vi "THz_TimeDelay.vi"(8 "error in (no error)":errorcluster, 11 "Transport":refnum<class "Transport.lvclass">) -> (0 "error out":errorcluster, 3 "Transport out":refnum<class "Transport.lvclass">)   [LabVIEW 2019, in "Transport.lvclass"]
uses:
  Transport.lvclass
  Control Experiment/Control Experiment.lvclass
  <vilib>/measure/NI_MAPro.lvlib
  <vilib>/PRIrvin/XY Utilities/xy_utilities.lvlib
  <vilib>/PRIrvin/XY Utilities/subVIs/Waveform to XY (single).vi
  <vilib>/PRIrvin/XY Utilities/subVIs/Get X and Y (single).vi
  <vilib>/measure/maspectr.llb/FFT Power Spectrum and PSD for 1 Chan.vi
  <userlib>/_MGI/Timing/MGI Wait/MGI Wait (U32).vi
  <vilib>/Waveform/WDTOps.llb/WDT Append Waveforms DBL.vi
  <userlib>/LevyLab/Lockin-Multichannel/Instrument.Lockin/Instrument.Lockin.lvclass
  <userlib>/LevyLab/Instrument Framework/Instrument Types/Cryostat/Instrument.Cryostat.lvclass
  <userlib>/LevyLab/Instrument Framework/Instrument Types/Delay Line/Instrument.DelayLine.lvclass
  <userlib>/LevyLab/Instrument Framework/Instrument Types/Lockin/Instrument.LockinAPI.lvclass
  89c60be8-115d-42a4-a854-67badb4f6eec.vi
  C:/Program Files/National Instruments/LabVIEW 2019/user.lib/LevyLab/Instrument Framework/Instrument Types/Lockin/Instrument.LockinAPI.lvclass
  <vilib>/measure/maresamp.llb/Resample Pair of Arrays (single shot).vi
panel:
  out "Horizontal Progress Bar":dbl(slide)=0.5013000000000001 scale=-0.5..0.5
  out "Signal vs Time":T1(graph)
  out "Delay vs Time":cluster{"Time":dbl[], "Delay":dbl[]}(graph)
  out "Power Spectrum":cluster{"f0":dbl, "df":dbl, "magnitude":dbl[]}[](graph) caption="Power spectrum of time domain signal"
  in  "stop":bool
  out "Experiment Comments":string="describe only the experiment you're doing right now"
  out "Experiment Folder":string="05 - folder name"
  out "Delay (ps)":dbl
  out "Elapsed Time (s)":u32
  out "T (mK)":dbl
  out "Refresh Time (ms)":u32
  in  "Sweep Time (s)":dbl=10.0 format="%#_3p"
  in  "Initial Wait (s)":u32=1
  in  "Delay End (ps)":dbl=0.5
  in  "Delay Start (ps)":dbl=-0.5
  in  "Fs (S/s)":dbl=1000.0 min=1000.0 max=204800.0 format="%#_13g"
  in  "Lockin Refresh (s)":dbl=2.0
  in  "Timeout (ms)":i32=1000
  out "Current State":string="Exit"
  # "Start"
  # "End"
  # "*Change these values in Transport Server"
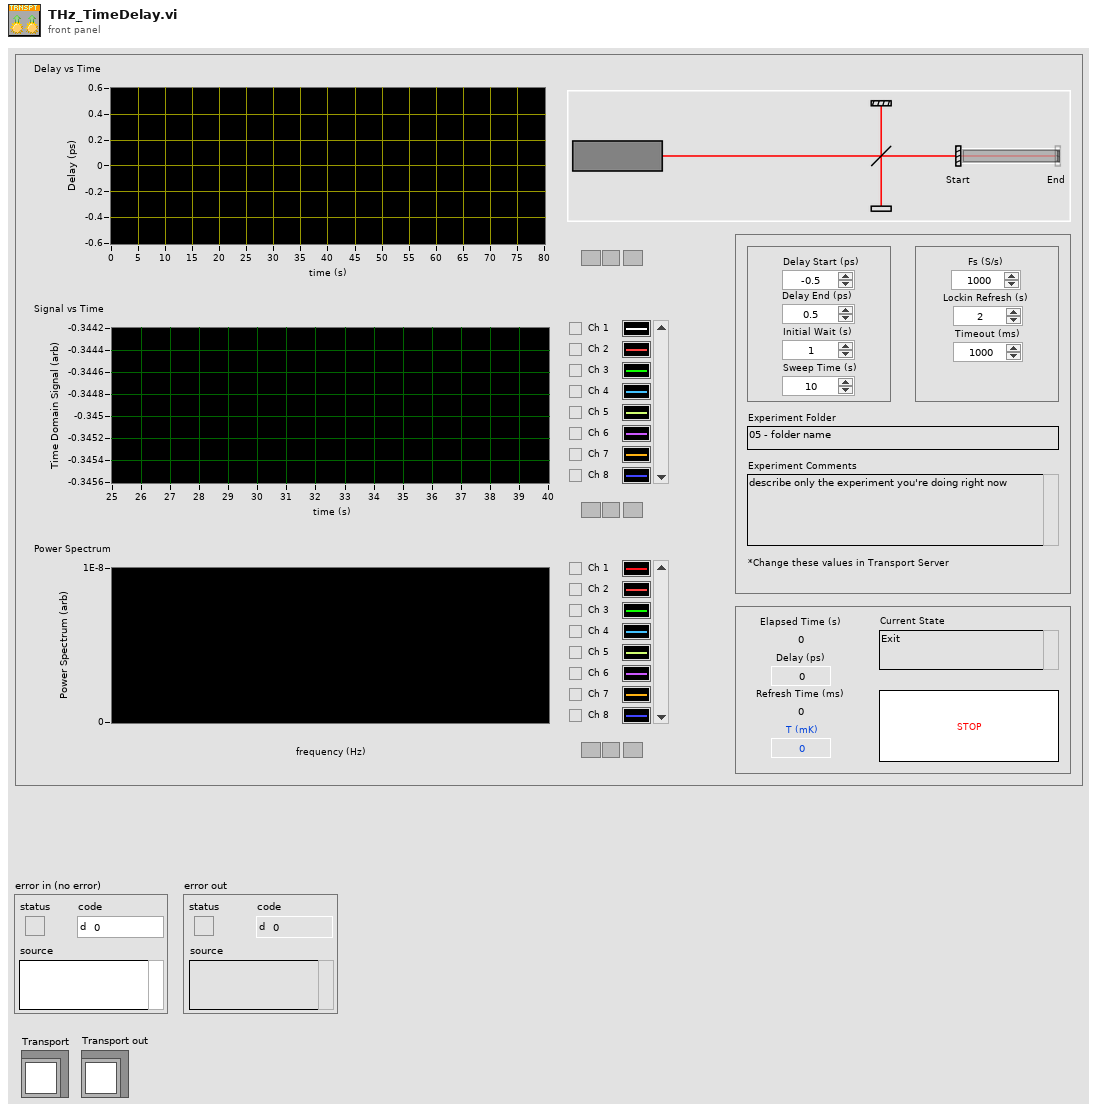
[diagram p1: front panel]
types:
  T1 = cluster{"Delay Start (ps)":dbl, dbl, "Y":dbl[]}[]
  T2 = enum32{"Invalid", "Standard", "Closed", "Hidden", "Minimized", "Maximized"}
  T3 = enum32{"invalid app kind", "Development System", "Run Time System", "Student Edition", "Embedded LabVIEW", "Evaluation", "Custom"}
  T4 = typedef "Control Experiment.lvclass/Instrument Classes--cluster.ctl" = cluster{"DAQ":refnum<class "Instrument.LockinAPI.lvclass">, "Amplifier":refnum<class "Instrument.Amplifier.lvclass">, "Temperature":refnum<class "Instrument.Cryostat.lvclass">, "Magnet":refnum<class "Instrument.Cryostat.lvclass">, "Rotator":refnum<class "Instrument.Cryostat.lvclass">, "Level":refnum<class "Instrument.Cryostat.lvclass">, "Capacitance":refnum<class "Instrument.CBridge.lvclass">, "Delay Line":refnum<class "Instrument.DelayLine.lvclass">, "Strain Cell":refnum<class "Instrument.Strain.lvclass">, "VNA":refnum<class "Instrument.VNA.lvclass">, "Source":refnum<class "Instrument.VSource.lvclass">}
  T5 = cluster{"Core":cluster{"Current VI Reference":refnum<vi>, "Close Panel on Exit?":bool}, "Transport":refnum<class "Transport.lvclass">, "C.E.":refnum<class "Control Experiment.lvclass">, "Instruments":T4, "Elapsed Time":dbl[], "Absolute Time":dbl[], "Temperature":dbl, "Magnet":dbl, "Delay":dbl[], "AI Waveform (s)":waveform(dbl)[], "AI Waveform (ps)":waveform(dbl)[], "t0":timestamp, "Sweep Value":dbl[], "ms [0]":u32, "ms [i]":u32, "Delay Range (ps)":dbl, "Delay Speed (ps/s)":dbl, "reset":bool, "delay line finish?":bool, "Execution:State":enum32{"Bad", "Idle", "Run top level", "Running"}}
  T6 = enum32{"Bad", "Idle", "Run top level", "Running"}
  T7 = cluster{"Current VI Reference":refnum<vi>, "Close Panel on Exit?":bool}
  T8 = typedef "Instrument.LockinAPI.lvclass/LockinAPI.Sampling.Sampling--Cluster.ctl" = cluster{"Fs":dbl, "#s":i32}
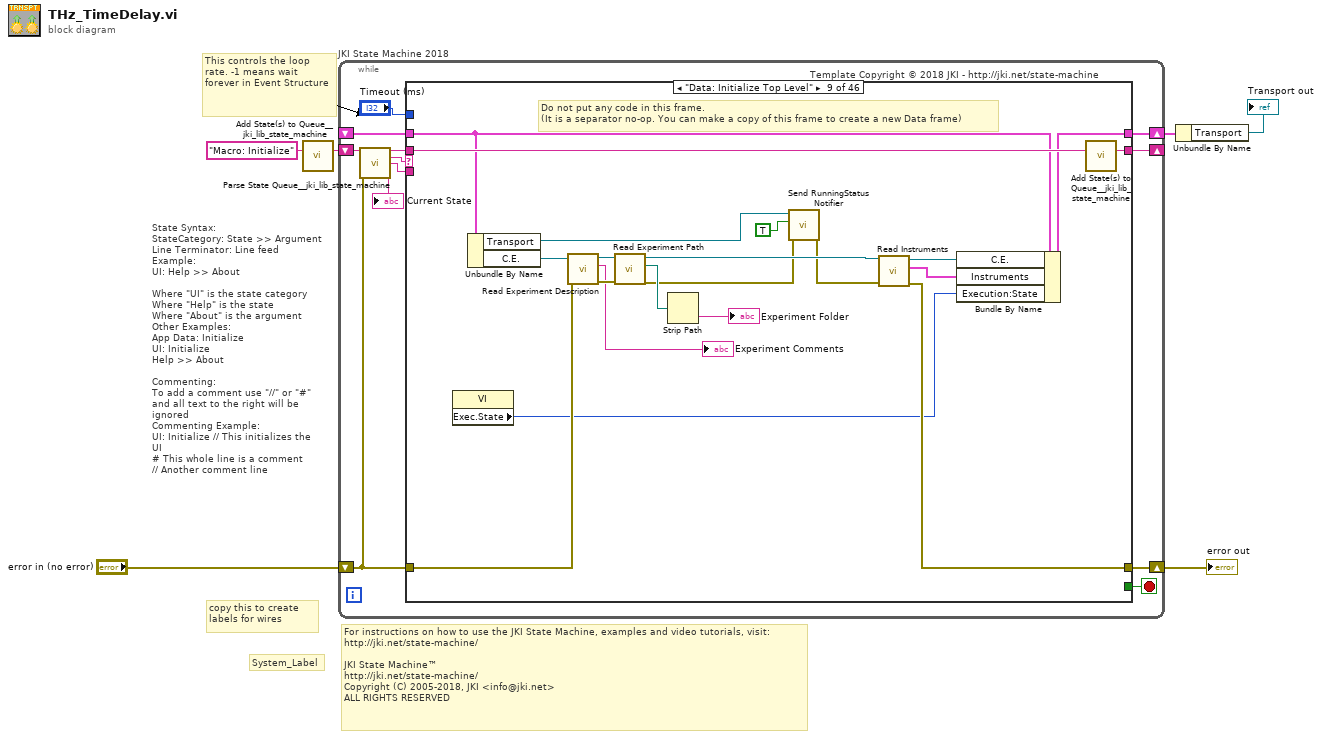
[diagram p0: block diagram]
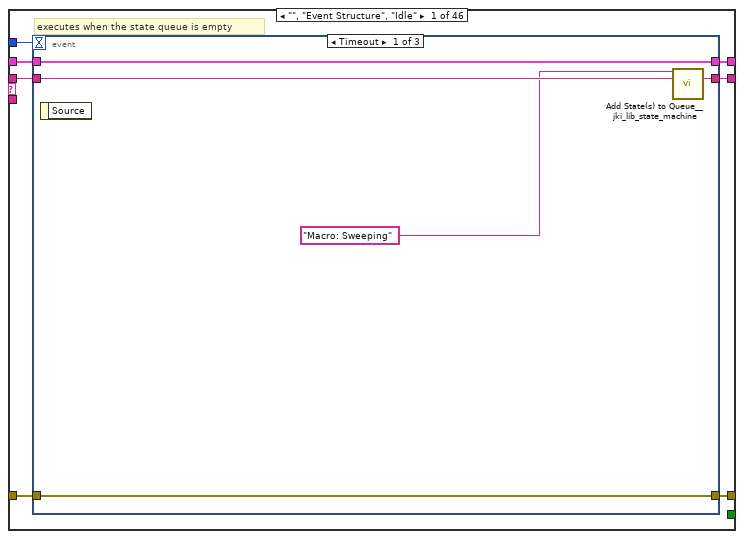
[diagram p2: hidden frame]
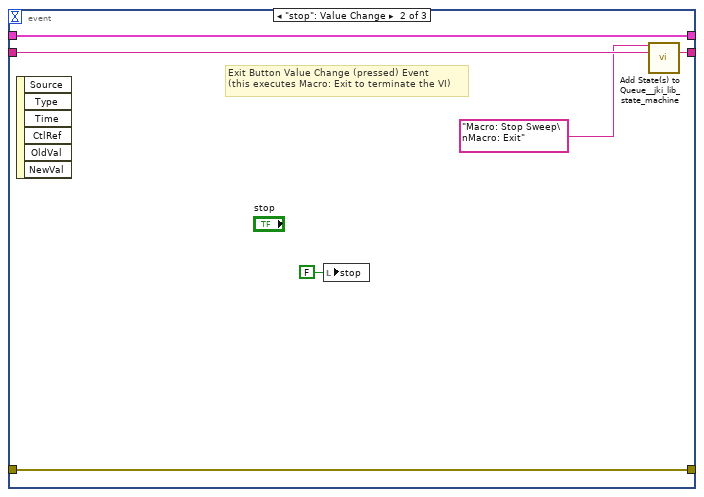
[diagram p3: hidden frame]
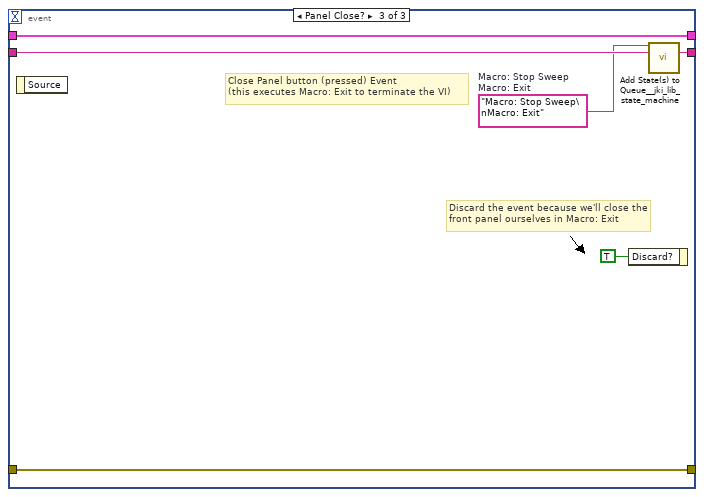
[diagram p4: hidden frame]
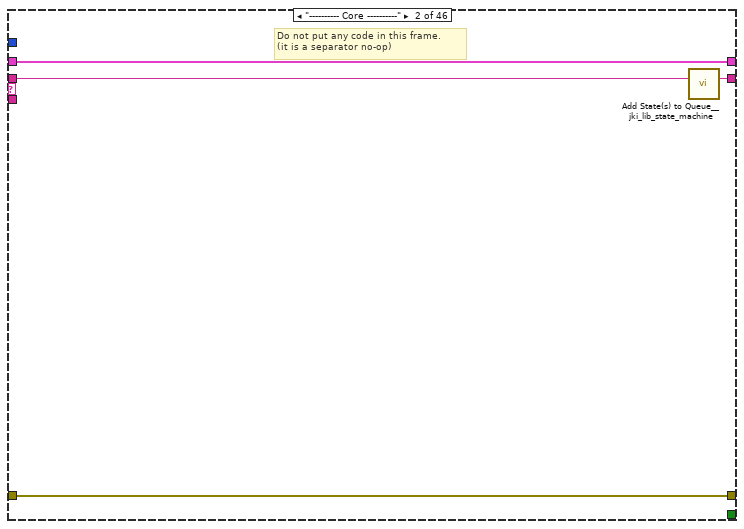
[diagram p5: hidden frame]
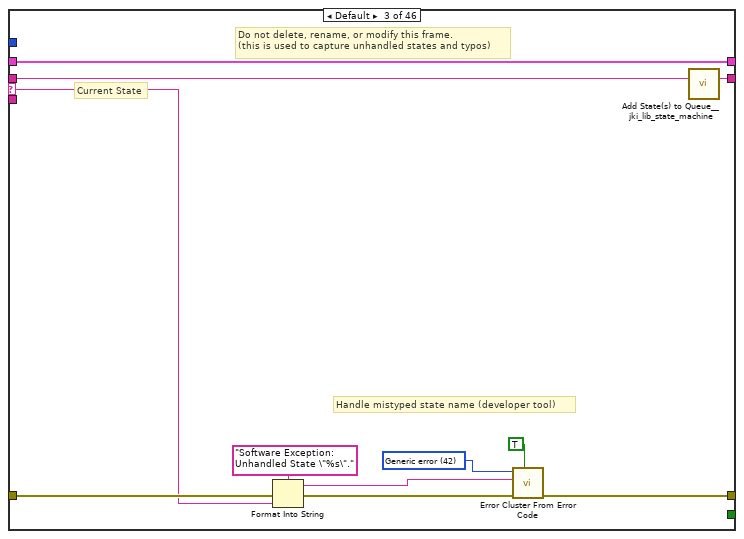
[diagram p6: hidden frame]
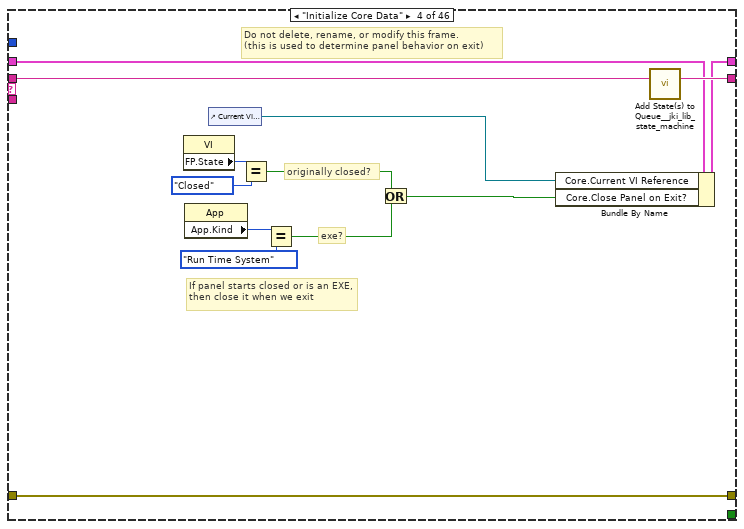
[diagram p7: hidden frame]
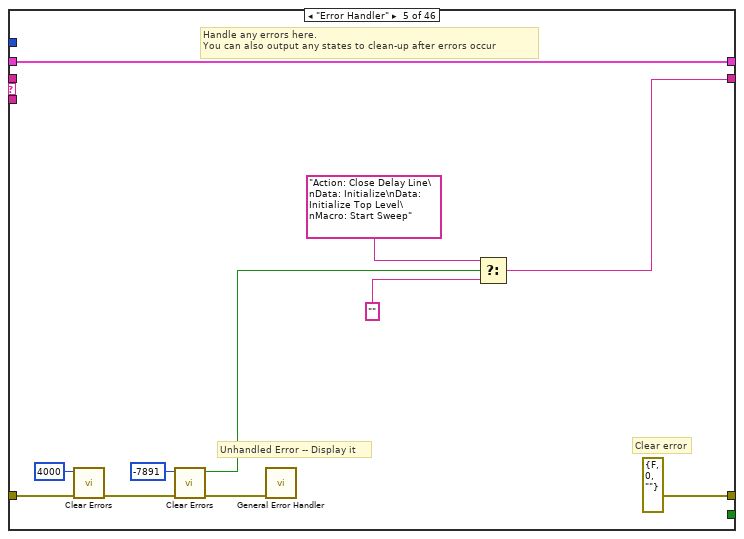
[diagram p8: hidden frame]
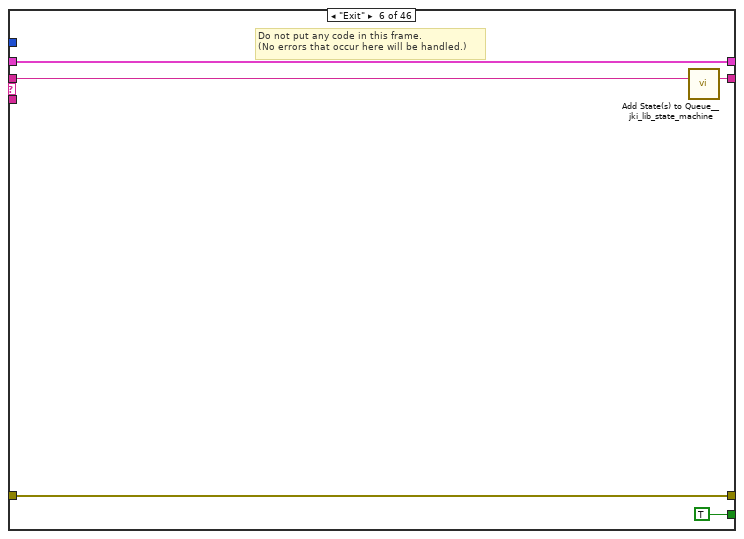
[diagram p9: hidden frame]
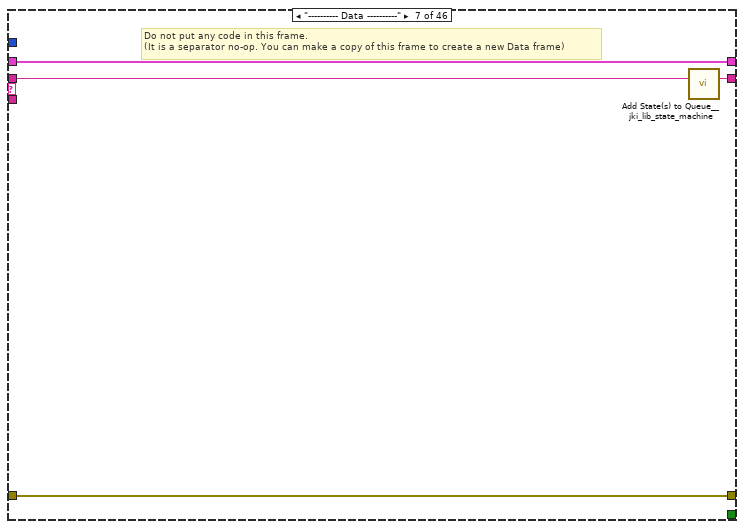
[diagram p10: hidden frame]
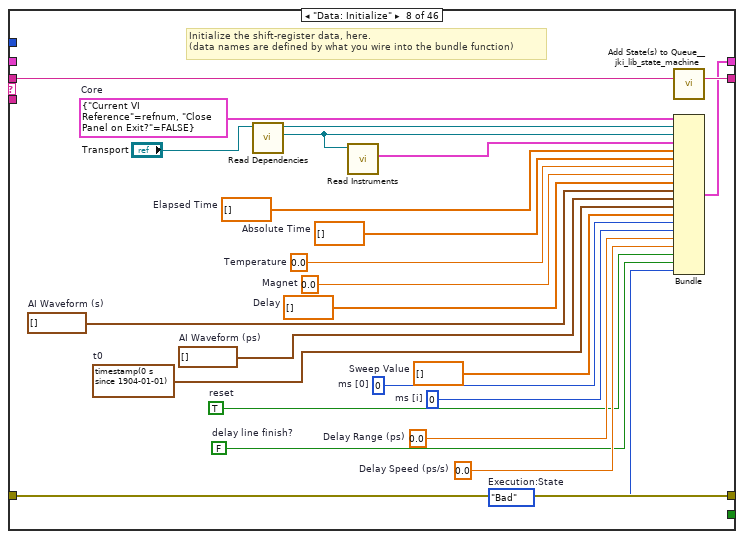
[diagram p11: hidden frame]
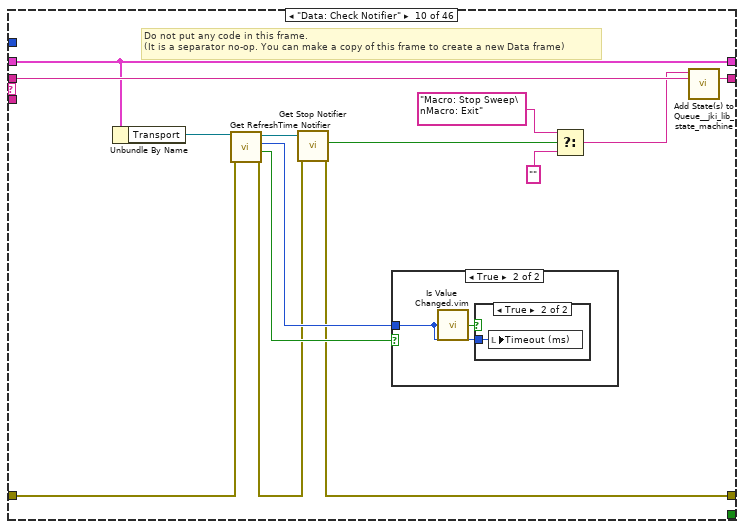
[diagram p12: hidden frame]
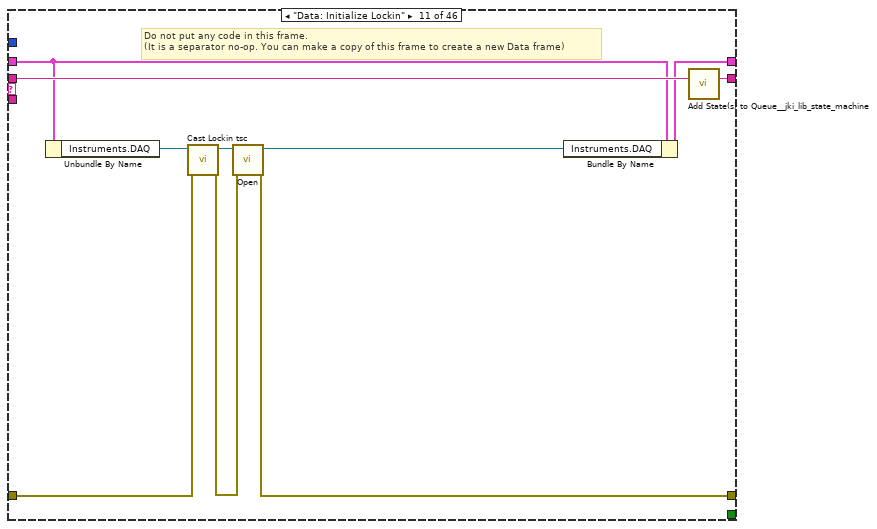
[diagram p15: hidden frame]
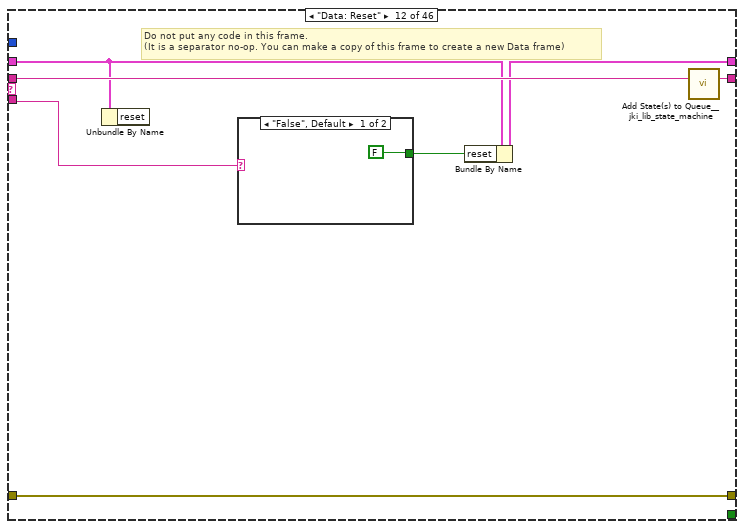
[diagram p16: hidden frame]
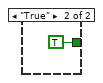
[diagram p17: hidden frame]
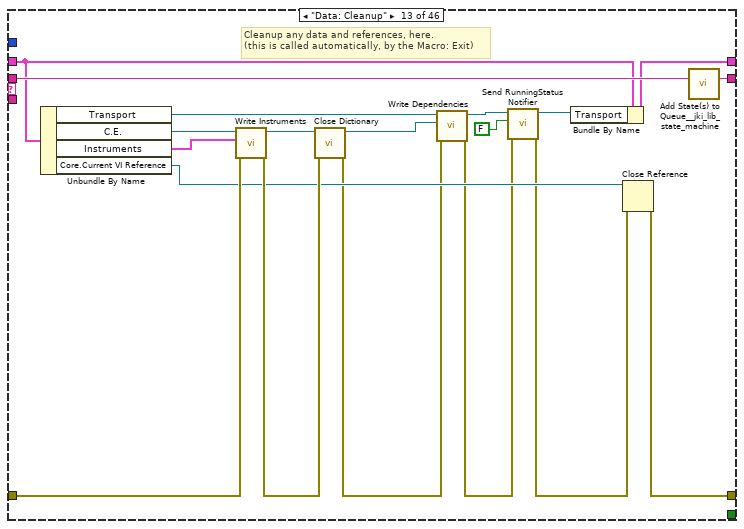
[diagram p18: hidden frame]
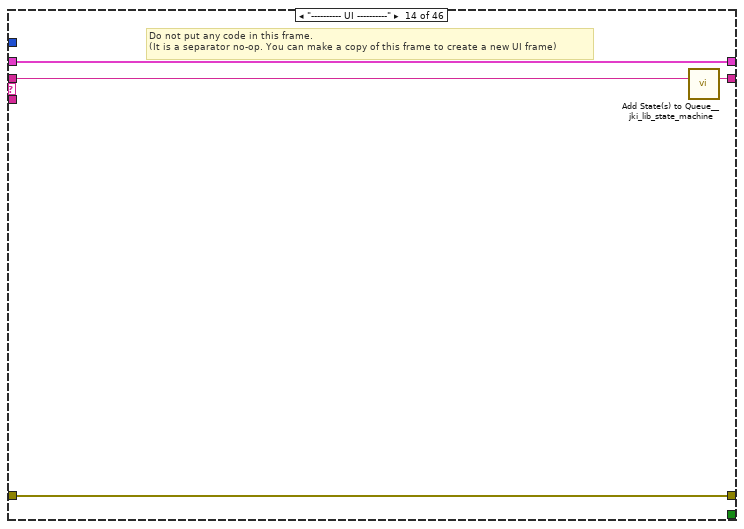
[diagram p19: hidden frame]
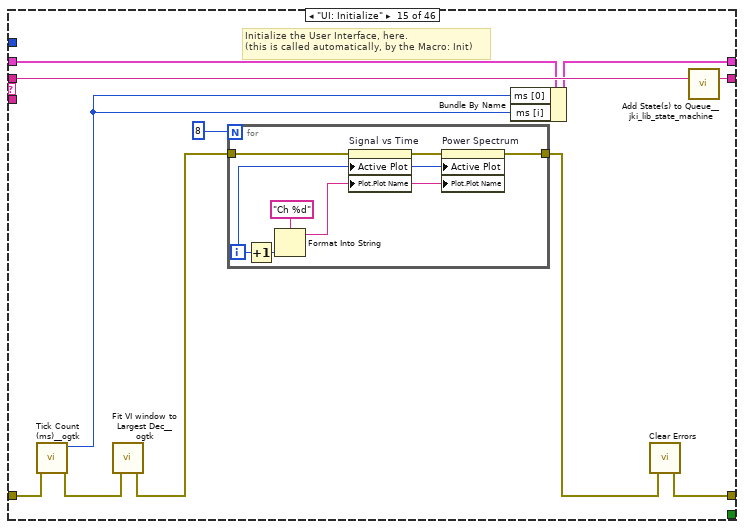
[diagram p20: hidden frame]
diagram:
  # "For instructions on how to use the JKI State Machine, examples and video tutorials, visit:\nhttp://jki.net/state-machine/\n\nJKI State Machine™\nhttp://jki.net/state-machine/\nCopyright (C) 2005-2018, JKI <info@jki.net>\nALL RIGHTS RESERVED"
  # "State Syntax:\nStateCategory: State >> Argument\nLine Terminator: Line feed\nExample:\nUI: Help >> About\n\nWhere \"UI\" is the state category\nWhere \"Help\" is the state\nWhere \"About\" is the argument\nOther Examples:\nApp Data: Initialize\nUI: Initialize\nHelp >> About\n\nCommenting:\nTo add a comment use \"//\" or \"#\" and all text to the right will be ignored\nCommenting Example:\nUI: Initialize // This initializes the UI\n# This whole line is a comment\n// Another comment line"
  # "copy this to create labels for wires"
  # "This controls the loop rate. -1 means wait forever in Event Structure"
  # "System_Label"
  n1 = call <vilib>:"Add State(s) to Queue__jki_lib_state_machine.vi"("State(s) in (\"\")"="Macro: Initialize") -> ("States Out"=w6:string)  [unwired: 14 in]
  n2 = while "JKI State Machine 2018" {
    shift-right: [w11] -> w4
    shift-left: _ -> [w10]
    shift-right: [w14] -> w3
    shift-left: "error in (no error)" -> [w8]
    shift-right: [w13] -> _
    shift-left: w6 -> [w15]
    stop <- w12 stop-if-true
    # "Template Copyright © 2018 JKI - http://jki.net/state-machine"
    n3 = call <vilib>:"Parse State Queue__jki_lib_state_machine.vi"("State Queue"=w15, "Error In (no error)"=w8) -> ("Remaining States"=w17:string, "Current State"=w7:string, "Arguments"=w16:string)  [unwired: 11 in]
    "Current State" <- w7
    n4 = case shown="\"Data: Initialize Top Level\"" w7 {
      selector: w7 -> [_ _ w46 _ _ _ _ _ _ _ _ _ _ _ _ _ _ _ _ _ _ _ _ _ _ _ _ _ _ _ _ _ _ _ _ _ _ _ _ _ _ _ _ _ _ _]
      tunnel: w17 -> [w24 w45 w50 w69 _ w85 w89 w114 w134 w148 w161 w168 w189 w193 w204 w217 w233 w256 w274 w281 w350 w358 w363 w368 w373 w383 w387 w401 w409 w413 w421 w426 w445 w454 w479 w498 w510 w514 w527 w586 w608 w626 w630 w634 w648 w693]
      tunnel: w16 -> [_ _ _ _ _ _ _ _ _ _ _ w163 _ _ _ w212 _ _ _ w275 _ _ _ _ _ _ _ _ _ _ _ _ _ w452 _ w495 _ _ w517 _ _ _ _ _ _ _]
      tunnel: w10 -> [w22 w42 w48 w62 w79 w83 w86 _ w126 w136 w157 w165 w187 w190 w200 w215 w224 w246 w269 w277 w347 w356 w359 w365 w370 w380 w384 w388 w407 w411 w419 w423 w442 w448 w465 w487 w505 w511 w525 w582 w605 w624 w627 w631 w638 w691]
      tunnel: [w21 w43 w52 w66 errorcluster {"status"=FALSE, "code"=0, "source"=""} ("error out") w82 w87 w111 w127 w138 w156 w166 w176 w191 w194 w213 w230 w248 w264 w278 w348 w355 w361 w366 w371 w381 w385 w393 w405 w410 w414 w424 w443 w449 w477 w490 w506 w512 w521 w576 w600 w615 w628 w632 w644 w690] -> w14
      tunnel: w8 -> [w20 w43 w51 w66 w77 w82 w87 w111 w128 w137 w152 w166 w181 w191 w201 w214 w230 w249 w271 w279 w348 w355 w361 w366 w371 w381 w385 w397 w406 w410 w414 w424 w443 w450 w469 w491 w507 w512 w518 w583 w601 w616 w628 w632 w643 w690]
      tunnel: [w23 w44 w49 w68 w74 w84 w88 w113 w133 w147 w160 w167 w188 w192 w203 w216 w232 w255 w273 w280 w349 w357 w362 w367 w372 w382 w386 w400 w408 w412 w420 w425 w444 w453 w478 w497 w509 w513 w526 w585 w607 w625 w629 w633 w647 w692] -> w13
      tunnel: [_ _ _ _ _ TRUE _ _ _ _ _ _ _ _ _ _ _ _ _ _ _ _ _ _ _ _ _ _ _ _ _ _ _ _ _ _ _ _ _ _ _ _ _ _ _ _] -> w12
      tunnel: [w19 w42 w48 w67 w79 w83 w86 w112 w125 w136 w158 w164 w186 w190 w199 w215 w223 w246 w268 w277 w347 w356 w359 w365 w370 w380 w384 w399 w407 w411 w419 w423 w442 w446 w464 w488 w503 w511 w524 w581 w606 w623 w627 w631 w637 w691] -> w11
      tunnel: "Timeout (ms)" -> [w18 _ _ _ _ _ _ _ _ _ _ _ _ _ _ _ _ _ _ _ _ _ _ _ _ _ _ _ _ _ _ _ _ _ _ _ _ _ _ _ _ _ _ _ _ _]
      frame "", "Event Structure", "Idle" {
        # "executes when the state queue is empty"
        n5 = event shown="[0] Timeout" {
          selector: _ -> [_ _ _]
          dyn-events: _ -> [_ _ _]
          timeout: w18 -> [_ _ _]
          tunnel: w24 -> [w29 w35 w41]
          tunnel: [w28 w34 w40] -> w23
          tunnel: w22 -> [w26 w32 w38]
          tunnel: [w27 w33 w39] -> w21
          tunnel: w20 -> [w27 w33 w39]
          tunnel: [w26 w32 w38] -> w19
          event Timeout {
            n6 = event-data() -> ()  [unwired: 1 in, 1 out]
            n7 = call <vilib>:"Add State(s) to Queue__jki_lib_state_machine.vi"("State(s) in Front (\"\")"="Macro: Sweeping" ("State(s) in Front (\"\")"), "State(s) in (\"\")"=w29) -> ("States Out"=w28:string)  [unwired: 13 in]
          }
          event "stop": Value Change {
            # "Exit Button Value Change (pressed) Event\n(this executes Macro: Exit to terminate the VI)"
            n8 = event-data() -> ()  [unwired: 1 in, 6 out]
            n9 = local write "stop"(FALSE ("stop")) -> ()
            n10 = call <vilib>:"Add State(s) to Queue__jki_lib_state_machine.vi"("State(s) in Front (\"\")"="Macro: Stop Sweep\nMacro: Exit", "State(s) in (\"\")"=w35) -> ("States Out"=w34:string)  [unwired: 13 in]
          }
          event Panel Close? {
            w37 = "Macro: Stop Sweep\nMacro: Exit"  # Macro: Stop Sweep Macro: Exit
            # "Discard the event because we'll close the front panel ourselves in Macro: Exit"
            # "Close Panel button (pressed) Event\n(this executes Macro: Exit to terminate the VI)"
            n11 = event-data() -> ()  [unwired: 1 in, 1 out]
            n12 = event-data("Discard?"=TRUE) -> ()  [unwired: 1 in, 1 out]
            n13 = call <vilib>:"Add State(s) to Queue__jki_lib_state_machine.vi"("State(s) in Front (\"\")"=w37, "State(s) in (\"\")"=w41) -> ("States Out"=w40:string)  [unwired: 13 in]
          }
        }
      }
      frame "---------- Core ----------" {
        # "Do not put any code in this frame.\n(it is a separator no-op)"
        n14 = call <vilib>:"Add State(s) to Queue__jki_lib_state_machine.vi"("State(s) in (\"\")"=w45) -> ("States Out"=w44:string)  [unwired: 14 in]
      }
      frame Default {
        w55 = 42 items=["No error", "Argument error", "Memory is full", "Out of zone", "End of file", "File already open", "Generic file I/O error", "File not found", "File permission error", "Disk is full", "Duplicate path", "Too many files open", "System feature not enabled", "Resource file not found", "Cannot add resource", "Resource not found", "Image not found", "Image memory error", "Pen does not exist", "Config type invalid", "Config token not found", "Config parse error", "Config memory error", "Bad external code format", "Bad external code offset", "External code not present", "Null window", "Destroy window error", "Null menu", "Print aborted", "Bad print record", "Print driver error", "Windows error during printing", "Memory error during printing", "Print dialog error", "Generic print error", "Invalid device refnum", "Device not found", "Device parameter error", "Device unit error", "Cannot open device", "Device call aborted", "Generic error", "Cancelled by user", "Object ID too low", "Object ID too high", "Object not in heap", "Unknown heap", "Unknown object (invalid DefProc)", "Unknown object (DefProc not in table)", "Message out of range", "Invalid (null) method", "Unknown message", "Manager call not supported", "Bad address", "Network operation in progress", "Network operation timed out", "Connection is busy", "Network attribute not supported", "Network error", "Address in use", "System out of memory", "Connection aborted", "Connection refused", "Not connected", "Already connected", "Connection closed", "Initialization error (interapplication manager)", "Bad occurrence", "Wait on unbound occurrence handler", "Occurrence queue overflow", "Datalog type conflict", "Unused", "Unrecognized type (interapplication manager)", "Memory corrupt", "Failed to make temporary DLL", "Old CIN version", "Drag socket not found", "Failed to load drop-object", "Failed to register OLE object", "Failed to release OLE object", "Format specifier type mismatch", "Unknown format specifier", "Too few format specifiers", "Too many format specifiers", "Scan failed", "Newer CIN version", "Error converting to variant", "Runtime menu error", "Password tampered", "Variant attribute not found", "Incompatible variant data type", "Event data is not available", "Event Store is not present", "Occurrence is not found", "Event Queue is not created", "Event info is not available", "Refnum passed is NULL", "Error retrieving Class GUID", "Error retrieving CoClass GUID", "Error retrieving TypeLib GUID.", "Bad built application magic bytes.", "Specific driver is different from the specific driver associated with the Logical Name.", "There is no session opened to the class driver.", "Max Error", "MAX - Error with config objects", "MAX - Error loading configuration", "MAX - Group not supported"]
        # "Current State"
        # "Do not delete, rename, or modify this frame.\n(this is used to capture unhandled states and typos)"
        # "Handle mistyped state name (developer tool)"
        n15 = Format Into String(format string="Software Exception: Unhandled State \"%s\"." ("message"), error in=w51, w46) -> (resulting string=w54:string, error out=w53:errorcluster)  [unwired: 1 in]
        n16 = call <vilib>:"Error Cluster From Error Code.vi"("show call chain? (False)"=TRUE, "error in (no error)"=w53, "error message (\"\")"=w54, "error code (0)"=w55) -> ("error out"=w52:errorcluster)  [unwired: 5 in]
        n17 = call <vilib>:"Add State(s) to Queue__jki_lib_state_machine.vi"("State(s) in (\"\")"=w50) -> ("States Out"=w49:string)  [unwired: 14 in]
      }
      frame "Initialize Core Data" {
        # "Do not delete, rename, or modify this frame.\n(this is used to determine panel behavior on exit)"
        # "originally closed?"
        # "exe?"
        # "If panel starts closed or is an EXE, then close it when we exit"
        n18 = property class="VI"() -> ("FP.State"=w59:T2)  [unwired: 2 in, 2 out]
        n19 = property class="App"() -> ("App.Kind"=w65:T3)  [unwired: 2 in, 2 out]
        n20 = control-ref of="Current VI Reference"() -> (w60:refnum<vi>)
        n21 = Equal?(x=w59, y=T2."Closed" ("Front Panel Window:State")) -> (x = y?=w57:bool)
        n22 = Equal?(x=w65, y=T3."Run Time System" ("Application:Kind")) -> (x = y?=w63:bool)
        n23 = Or(x=w57, y=w63) -> (x .or. y?=w61:bool)
        n24 = Bundle By Name(cluster=w62, "Core.Current VI Reference"=w60, "Core.Close Panel on Exit?"=w61) -> (w67:T5)
        n25 = call <vilib>:"Add State(s) to Queue__jki_lib_state_machine.vi"("State(s) in (\"\")"=w69) -> ("States Out"=w68:string)  [unwired: 14 in]
      }
      frame "Error Handler" {
        # "Unhandled Error -- Display it"
        # "Handle any errors here.\nYou can also output any states to clean-up after errors occur"
        # "Clear error"
        n26 = call <vilib>:"Clear Errors.vi"("error in (no error)"=w77, "specific error code to clear (0: all)"=4000) -> ("error out"=w72:errorcluster)  [unwired: 4 in, 1 out]
        n27 = call <vilib>:"Clear Errors.vi"("error in (no error)"=w72, "specific error code to clear (0: all)"=-7891) -> ("error out"=w71:errorcluster, "specific error cleared?"=w70:bool)  [unwired: 4 in]
        n28 = call <vilib>:"General Error Handler.vi"("error in (no error)"=w71) -> ()  [unwired: 10 in, 5 out]
        n29 = Select(t="Action: Close Delay Line\nData: Initialize\nData: Initialize Top Level\nMacro: Start Sweep", s=w70, f="") -> (s? t:f=w74:string)
      }
      frame "Exit" {
        # "Do not put any code in this frame.\n(No errors that occur here will be handled.)"
        n30 = call <vilib>:"Add State(s) to Queue__jki_lib_state_machine.vi"("State(s) in (\"\")"=w85) -> ("States Out"=w84:string)  [unwired: 14 in]
      }
      frame "---------- Data ----------" {
        # "Do not put any code in this frame.\n(It is a separator no-op. You can make a copy of this frame to create a new Data frame)"
        n31 = call <vilib>:"Add State(s) to Queue__jki_lib_state_machine.vi"("State(s) in (\"\")"=w89) -> ("States Out"=w88:string)  [unwired: 14 in]
      }
      frame "Data: Initialize" {
        w94 = T6."Bad"  # Execution:State
        w95 = waveform(dbl)[] []  # AI Waveform (ps)
        w96 = FALSE  # delay line finish?
        w97 = TRUE  # reset
        w102 = dbl[] []  # Absolute Time
        w98 = waveform(dbl)[] []  # AI Waveform (s)
        w104 = timestamp(0 s since 1904-01-01)  # t0
        w105 = 0.0  # Delay Speed (ps/s)
        w99 = dbl[] []  # Delay
        w106 = 0.0  # Delay Range (ps)
        w107 = dbl[] []  # Sweep Value
        w108 = u32 0  # ms [i]
        w109 = u32 0  # ms [0]
        w103 = dbl[] []  # Elapsed Time
        w100 = 0.0  # Magnet
        w101 = 0.0  # Temperature
        w110 = T7 {"Current VI Reference"=refnum, "Close Panel on Exit?"=FALSE}  # Core
        # "Initialize the shift-register data, here.\n(data names are defined by what you wire into the bundle function)"
        n32 = call "Read Dependencies.vi"("Transport"="Transport") -> ("C.E."=w91:refnum<class "Control Experiment.lvclass">, "Transport"=w92:refnum<class "Transport.lvclass">)  [unwired: 8 in, 1 out]
        n33 = call "Read Instruments.vi"("Control Experiment in"=w91) -> ("Instruments"=w90:T4)  [unwired: 8 in, 2 out]
        n34 = call <vilib>:"Add State(s) to Queue__jki_lib_state_machine.vi"("State(s) in (\"\")"=w114) -> ("States Out"=w113:string)  [unwired: 14 in]
        n35 = Bundle("Core"=w110, "Transport"=w92, "C.E."=w91, "Instruments"=w90, "Elapsed Time"=w103, "Absolute Time"=w102, "Temperature"=w101, "Magnet"=w100, "Delay"=w99, "AI Waveform (s)"=w98, "AI Waveform (ps)"=w95, "t0"=w104, "Sweep Value"=w107, "ms [0]"=w109, "ms [i]"=w108, "Delay Range (ps)"=w106, "Delay Speed (ps/s)"=w105, "reset"=w97, "delay line finish?"=w96, "Execution:State"=w94) -> (w112:T5)  [unwired: 1 in]
      }
      frame "Data: Initialize Top Level" {
        # "Do not put any code in this frame.\n(It is a separator no-op. You can make a copy of this frame to create a new Data frame)"
        n36 = property class="VI"() -> ("Exec.State"=w123:T6)  [unwired: 2 in, 2 out]
        n37 = Unbundle By Name(w126) -> ("Transport"=w122:refnum<class "Transport.lvclass">, "C.E."=w129:refnum<class "Control Experiment.lvclass">)
        n38 = call "Read Experiment Description.vi"("error in (no error)"=w128, "Control Experiment in"=w129) -> ("error out"=w120:errorcluster, "Experiment Description"=→"Experiment Comments":string, "Control Experiment out"=w119:refnum<class "Control Experiment.lvclass">)  [unwired: 7 in]
        n39 = call "Read Experiment Path.vi"("error in (no error)"=w120, "Control Experiment in"=w119) -> ("error out"=w117:errorcluster, "Experiment Path"=w121:path, "Control Experiment out"=w131:refnum<class "Control Experiment.lvclass">)  [unwired: 7 in]
        n40 = Strip Path(path=w121) -> (name=→"Experiment Folder":string)  [unwired: 1 out]
        n41 = call "Send RunningStatus Notifier.vi"("error in (no error)"=w117, "Running?"=TRUE, "Transport in"=w122) -> ("error out"=w130:errorcluster)  [unwired: 7 in, 1 out]
        n42 = call "Read Instruments.vi"("error in (no error)"=w130, "Control Experiment in"=w131) -> ("error out"=w127:errorcluster, "Instruments"=w132:T4, "Control Experiment out"=w124:refnum<class "Control Experiment.lvclass">)  [unwired: 7 in]
        n43 = Bundle By Name(cluster=w126, "C.E."=w124, "Instruments"=w132, "Execution:State"=w123) -> (w125:T5)
        n44 = call <vilib>:"Add State(s) to Queue__jki_lib_state_machine.vi"("State(s) in (\"\")"=w134) -> ("States Out"=w133:string)  [unwired: 14 in]
      }
      frame "Data: Check Notifier" {
        # "Do not put any code in this frame.\n(It is a separator no-op. You can make a copy of this frame to create a new Data frame)"
        n45 = Unbundle By Name(w136) -> ("Transport"=w143:refnum<class "Transport.lvclass">)
        n46 = call "Get RefreshTime Notifier.vi"("error in (no error)"=w137, "Transport in"=w143) -> ("error out"=w139:errorcluster, "valid?"=w140:bool, "RefreshTime (ms)"=w141:u32, "Transport out"=w142:refnum<class "Transport.lvclass">)  [unwired: 6 in]
        n47 = call "Get Stop Notifier.vi"("error in (no error)"=w139, "Transport in"=w142) -> ("error out"=w138:errorcluster, "Stop?"=w144:bool)  [unwired: 7 in, 1 out]
        n48 = case shown="True" w140 {
          tunnel: w141 -> [_ w149]
          frame False {
          }
          frame True {
            n49 = call "Is Value Changed.vim"("value"=w149) -> ("changed or first call?"=w150:bool)
            n50 = case shown="True" w150 {
              tunnel: w149 -> [_ w151]
              frame False {
              }
              frame True {
                n51 = local write "Timeout (ms)"(w151) -> ()
              }
            }
          }
        }
        n52 = Select(t="Macro: Stop Sweep\nMacro: Exit", s=w144, f="") -> (s? t:f=w135:string)
        n53 = call <vilib>:"Add State(s) to Queue__jki_lib_state_machine.vi"("State(s) in Front (\"\")"=w135, "State(s) in (\"\")"=w148) -> ("States Out"=w147:string)  [unwired: 13 in]
      }
      frame "Data: Initialize Lockin" {
        # "Do not put any code in this frame.\n(It is a separator no-op. You can make a copy of this frame to create a new Data frame)"
        n54 = Unbundle By Name(w157) -> ("Instruments.DAQ"=w155:refnum<class "Instrument.LockinAPI.lvclass">)
        n55 = call "Cast Lockin tsc.vi"("error in (no error)"=w152, "Instrument.LockinAPI in"=w155) -> ("error out"=w153:errorcluster, "Instrument.Lockin out"=w154:refnum<class "Instrument.Lockin.lvclass">)  [unwired: 8 in]
        n56 = call-dynamic "Open.vi"("error in (no error)"=w153, "Instrument.Lockin in"=w154) -> ("error out"=w156:errorcluster, "Instrument.Lockin out"=w159:refnum<class "Instrument.Lockin.lvclass">)  [unwired: 8 in]
        n57 = Bundle By Name(cluster=w157, "Instruments.DAQ"=w159) -> (w158:T5)
        n58 = call <vilib>:"Add State(s) to Queue__jki_lib_state_machine.vi"("State(s) in (\"\")"=w161) -> ("States Out"=w160:string)  [unwired: 14 in]
      }
      frame "Data: Reset" {
        # "Do not put any code in this frame.\n(It is a separator no-op. You can make a copy of this frame to create a new Data frame)"
        n59 = Unbundle By Name(w165) -> ()  [unwired: 1 out]
        n60 = case shown="\"False\", Default" w163 {
          tunnel: [FALSE ("reset") TRUE ("reset")] -> w162
          frame "False", Default {
          }
          frame "True" {
          }
        }
        n61 = Bundle By Name(cluster=w165, "reset"=w162) -> (w164:T5)
        n62 = call <vilib>:"Add State(s) to Queue__jki_lib_state_machine.vi"("State(s) in (\"\")"=w168) -> ("States Out"=w167:string)  [unwired: 14 in]
      }
      frame "Data: Cleanup" {
        # "Cleanup any data and references, here.\n(this is called automatically, by the Macro: Exit)"
        n63 = Unbundle By Name(w187) -> ("Transport"=w185:refnum<class "Transport.lvclass">, "C.E."=w184:refnum<class "Control Experiment.lvclass">, "Instruments"=w182:T4, "Core.Current VI Reference"=w179:refnum<vi>)
        n64 = call "Write Instruments.vi"("error in (no error)"=w181, "Instruments"=w182, "Control Experiment in"=w184) -> ("error out"=w180:errorcluster, "Control Experiment out"=w183:refnum<class "Control Experiment.lvclass">)  [unwired: 7 in]
        n65 = call "Close Dictionary.vi"("error in (no error)"=w180, "Control Experiment in"=w183) -> ("error out"=w177:errorcluster, "Control Experiment out"=w178:refnum<class "Control Experiment.lvclass">)  [unwired: 8 in]
        n66 = call "Write Dependencies.vi"("error in (no error)"=w177, "Control Experiment"=w178, "Transport in"=w185) -> ("error out"=w172:errorcluster, "Transport out"=w174:refnum<class "Transport.lvclass">)  [unwired: 7 in]
        n67 = call "Send RunningStatus Notifier.vi"("error in (no error)"=w172, "Running?"=FALSE, "Transport in"=w174) -> ("error out"=w171:errorcluster, "Transport out"=w173:refnum<class "Transport.lvclass">)  [unwired: 7 in]
        n68 = Bundle By Name(cluster=w187, "Transport"=w173) -> (w186:T5)
        n69 = Close Reference(reference=w179, error in (no error)=w171) -> (error out=w176:errorcluster)
        n70 = call <vilib>:"Add State(s) to Queue__jki_lib_state_machine.vi"("State(s) in (\"\")"=w189) -> ("States Out"=w188:string)  [unwired: 14 in]
      }
      frame "---------- UI ----------" {
        # "Do not put any code in this frame.\n(It is a separator no-op. You can make a copy of this frame to create a new UI frame)"
        n71 = call <vilib>:"Add State(s) to Queue__jki_lib_state_machine.vi"("State(s) in (\"\")"=w193) -> ("States Out"=w192:string)  [unwired: 14 in]
      }
      frame "UI: Initialize" {
        # "Initialize the User Interface, here.\n(this is called automatically, by the Macro: Init)"
        n72 = call <userlib>:"Tick Count (ms)__ogtk.vi"("error in (no error)"=w201) -> ("error out"=w197:errorcluster, "millisecond timer value"=w198:u32)  [unwired: 9 in]
        n73 = call <userlib>:"Fit VI window to Largest Dec__ogtk.vi"("error in (no error)"=w197) -> ("error out"=w196:errorcluster)  [unwired: 5 in, 1 out]
        n74 = for {
          N: 8 -> [_]
          tunnel: w196 -> [w210]
          tunnel: [w206] -> w195
          i -> [w207]
          n75 = Increment(x=w207) -> (x+1=w209:i32)
          n76 = Format Into String(format string="Ch %d", w209) -> (resulting string=w205:string)  [unwired: 2 in, 1 out]
          n77 = property on="Signal vs Time" class="WFGraph (strict)"(error in=w210, "Active Plot"=w207, "Plot.Plot Name"=w205) -> (error out=w208:errorcluster)  [unwired: 1 in, 1 out]
          n78 = property on="Power Spectrum" class="WFGraph (strict)"(error in=w208, "Active Plot"=w207, "Plot.Plot Name"=w205) -> (error out=w206:errorcluster)  [unwired: 1 in, 1 out]
        }
        n79 = Bundle By Name(cluster=w200, "ms [0]"=w198, "ms [i]"=w198) -> (w199:T5)
        n80 = call <vilib>:"Clear Errors.vi"("error in (no error)"=w195) -> ("error out"=w194:errorcluster)  [unwired: 5 in, 1 out]
        n81 = call <vilib>:"Add State(s) to Queue__jki_lib_state_machine.vi"("State(s) in (\"\")"=w204) -> ("States Out"=w203:string)  [unwired: 14 in]
      }
      frame "UI: Cursor Set" {
        # "Argument"
        # "Set and Unset Cursor Busy.\n(Usage: \"UI: Cursor Set >> Busy|Idle\")"
        n82 = case shown="\"Idle\", Default" w212 {
          tunnel: w214 -> [w219 w221]
          tunnel: [w218 w220] -> w213
          frame "Idle", Default {
            n83 = call <vilib>:"Unset Busy.vi"("error in (no error)"=w219) -> ("error out"=w218:errorcluster)  [unwired: 10 in]
          }
          frame "Busy" {
            n84 = call <vilib>:"Set Busy.vi"("error in (no error)"=w221) -> ("error out"=w220:errorcluster)  [unwired: 9 in, 1 out]
          }
        }
        n85 = call <vilib>:"Add State(s) to Queue__jki_lib_state_machine.vi"("State(s) in (\"\")"=w217) -> ("States Out"=w216:string)  [unwired: 14 in]
      }
      frame "UI: Update Graphs" {
        # "Do not put any code in this frame.\n(It is a separator no-op. You can make a copy of this frame to create a new UI frame)"
        n86 = Unbundle By Name(w224) -> ("Elapsed Time"=w231:dbl[], "Delay"=w229:dbl[], "AI Waveform (s)"=w227:waveform(dbl)[], "Delay Speed (ps/s)"=w225:dbl)  [unwired: 1 out]
        n87 = Bundle("Elapsed Time"=w231, "Delay"=w229) -> (→"Delay vs Time":cluster{"Elapsed Time":dbl[], "Delay":dbl[]})  [unwired: 1 in]
        n88 = for {
          tunnel: w227 -> [w235] mode=indexing
          tunnel: [w237] -> w226 mode=indexing
          tunnel: w225 -> [w236]
          tunnel: [w234] -> w222 mode=indexing
          # "dt in ps"
          # "ps/s"
          # "dt in seconds"
          n89 = Unbundle By Name(w235) -> ("dt"=w241:dbl, "Y"=w239:dbl[])
          n90 = local read "Delay Start (ps)"() -> (w238:dbl)
          n91 = Multiply(x=w241, y=w236) -> (x*y=w240:dbl)
          n92 = Bundle By Name(cluster=w235, "dt"=w236) -> (w234:waveform(dbl))
          n93 = Bundle("Delay Start (ps)"=w238, w240, "Y"=w239) -> (w237:cluster{"Delay Start (ps)":dbl, dbl, "Y":dbl[]})  [unwired: 1 in]
        }
        "Signal vs Time" <- w226
        n94 = Bundle By Name(cluster=w224, "AI Waveform (ps)"=w222) -> (w223:T5)
        n95 = call <vilib>:"Add State(s) to Queue__jki_lib_state_machine.vi"("State(s) in (\"\")"=w233) -> ("States Out"=w232:string)  [unwired: 14 in]
      }
      frame "UI: Update Graphs Final" {
        # "Do not put any code in this frame.\n(It is a separator no-op. You can make a copy of this frame to create a new UI frame)"
        n96 = Unbundle By Name(w246) -> ("Absolute Time"=w244:dbl[], "Elapsed Time"=w251:dbl[], "Delay"=w245:dbl[], "AI Waveform (s)"=w242:waveform(dbl)[])
        n97 = Index Array(array=w242) -> (element=w254:waveform(dbl))  [unwired: 1 in]
        n98 = Bundle("Elapsed Time"=w251, "Delay"=w245) -> ()  [unwired: 1 in, 1 out]
        n99 = Unbundle By Name(w254) -> ("dt"=w253:dbl, "t0"=w252:timestamp)
        n100 = Bundle("Absolute Time"=w244, "Delay"=w245) -> (w243:cluster{"Absolute Time":dbl[], "Delay":dbl[]})  [unwired: 1 in]
        n101 = To Double Precision Float(number=w252) -> (double precision float=w250:dbl)
        n102 = call-poly <vilib>:"Resample Waveforms (single shot).vi"("XY-data in"=w243, "dt"=w253, "t0"=w250, "error in (no error)"=w249) -> ("resampled waveform out"=w247:waveform(dbl), "error out"=w248:errorcluster)  [unwired: 7 in, 3 out]
        n103 = for {
          tunnel: w247 -> [w261]
          tunnel: w242 -> [w260] mode=indexing
          tunnel: [w257] -> _ mode=indexing
          n104 = Unbundle By Name(w261) -> ("Y"=w259:dbl[])
          n105 = Unbundle By Name(w260) -> ("Y"=w258:dbl[])
          n106 = Bundle("Y"=w259, "Y"=w258) -> (w257:cluster{"Y":dbl[], "Y":dbl[]})  [unwired: 1 in]
        }
        n107 = call <vilib>:"Add State(s) to Queue__jki_lib_state_machine.vi"("State(s) in (\"\")"=w256) -> ("States Out"=w255:string)  [unwired: 14 in]
      }
      frame "UI: Update Timer" {
        n108 = Unbundle By Name(w269) -> ("ms [0]"=w270:u32)
        n109 = call <userlib>:"Tick Count (ms)__ogtk.vi"("error in (no error)"=w271) -> ("error out"=w265:errorcluster, "millisecond timer value"=w263:u32)  [unwired: 9 in]
        n110 = Subtract(x=w263, y=w270) -> (x-y=w267:u32)
        n111 = call <userlib>:"MGI Milliseconds Since Last Call.vi"("Error In"=w265) -> ("ms"=→"Refresh Time (ms)":u32, "Error Out"=w264:errorcluster)  [unwired: 5 in]
        n112 = Divide(x=w267, y=u32 1000 ("x")) -> (x/y=→"Elapsed Time (s)":dbl)
        n113 = Bundle By Name(cluster=w269, "ms [i]"=w263) -> (w268:T5)
        n114 = call <vilib>:"Add State(s) to Queue__jki_lib_state_machine.vi"("State(s) in (\"\")"=w274) -> ("States Out"=w273:string)  [unwired: 14 in]
      }
      frame "UI: Front Panel State" {
        # "Argument"
        # "Set Front Panel Open or Closed\n(Usage: \"UI: Front Panel State >> Open|Close\")"
        n115 = Unbundle By Name(w277) -> ("Core.Current VI Reference"=w276:refnum<vi>)
        n116 = case shown="\"Open\", \"Standard\", Default" w275 {
          tunnel: w279 -> [w287 w302 w313 w326 w339]
          tunnel: [w289 w303 w315 w328 w341] -> w278
          tunnel: w276 -> [w288 w300 w314 w327 w340]
          frame "Open", "Standard", Default {
            w282 = T2."Standard" ("State")
            n117 = property class="VI"(reference=w288, error in=w287) -> (reference out=w285:refnum<vi>, error out=w286:errorcluster, "FP.State"=w284:T2)
            n118 = Not Equal?(x=w284, y=w282) -> (x != y?=w283:bool)
            n119 = case shown="False" w283 {
              tunnel: [w293 w295] -> w289
              tunnel: w286 -> [w292 w295]
              tunnel: w285 -> [w291 _]
              tunnel: w282 -> [w290 _]
              frame True {
                n120 = invoke class="VI" method="FP.Open"(reference=w291, error in=w292, "Activate"=TRUE, "State"=w290) -> (error out=w293:errorcluster)  [unwired: 1 in, 4 out]
              }
              frame False {
              }
            }
          }
          frame "Close", "Closed" {
            n121 = property class="VI"(reference=w300, error in=w302) -> (reference out=w299:refnum<vi>, error out=w301:errorcluster, "FP.State"=w297:T2)
            n122 = Not Equal?(x=w297, y=T2."Closed" ("Front Panel Window:State")) -> (x != y?=w296:bool)
            n123 = case shown="True" w296 {
              tunnel: [w304 w307] -> w303
              tunnel: w301 -> [w304 w306]
              tunnel: w299 -> [_ w305]
              frame False {
              }
              frame True {
                n124 = invoke class="VI" method="FP.Close"(reference=w305, error in=w306) -> (error out=w307:errorcluster)  [unwired: 1 in, 2 out]
              }
            }
          }
          frame "Hidden", "Hide" {
            w308 = T2."Hidden" ("State")
            n125 = property class="VI"(reference=w314, error in=w313) -> (reference out=w311:refnum<vi>, error out=w312:errorcluster, "FP.State"=w310:T2)
            n126 = Not Equal?(x=w310, y=w308) -> (x != y?=w309:bool)
            n127 = case shown="True" w309 {
              tunnel: [w319 w320] -> w315
              tunnel: w312 -> [w318 w320]
              tunnel: w311 -> [w317 _]
              tunnel: w308 -> [w316 _]
              frame True {
                n128 = invoke class="VI" method="FP.Open"(reference=w317, error in=w318, "State"=w316) -> (error out=w319:errorcluster)  [unwired: 2 in, 4 out]
              }
              frame False {
              }
            }
          }
          frame "Minimize", "Minimized" {
            w321 = T2."Minimized" ("State")
            n129 = property class="VI"(reference=w327, error in=w326) -> (reference out=w324:refnum<vi>, error out=w325:errorcluster, "FP.State"=w323:T2)
            n130 = Not Equal?(x=w323, y=w321) -> (x != y?=w322:bool)
            n131 = case shown="True" w322 {
              tunnel: [w332 w333] -> w328
              tunnel: w325 -> [w331 w333]
              tunnel: w324 -> [w330 _]
              tunnel: w321 -> [w329 _]
              frame True {
                n132 = invoke class="VI" method="FP.Open"(reference=w330, error in=w331, "State"=w329) -> (error out=w332:errorcluster)  [unwired: 2 in, 4 out]
              }
              frame False {
              }
            }
          }
          frame "Maximize", "Maximized" {
            w334 = T2."Maximized" ("State")
            n133 = property class="VI"(reference=w340, error in=w339) -> (reference out=w337:refnum<vi>, error out=w338:errorcluster, "FP.State"=w336:T2)
            n134 = Not Equal?(x=w336, y=w334) -> (x != y?=w335:bool)
            n135 = case shown="True" w335 {
              tunnel: [w345 w346] -> w341
              tunnel: w338 -> [w344 w346]
              tunnel: w337 -> [w343 _]
              tunnel: w334 -> [w342 _]
              frame True {
                n136 = invoke class="VI" method="FP.Open"(reference=w343, error in=w344, "State"=w342) -> (error out=w345:errorcluster)  [unwired: 2 in, 4 out]
              }
              frame False {
              }
            }
          }
        }
        n137 = call <vilib>:"Add State(s) to Queue__jki_lib_state_machine.vi"("State(s) in (\"\")"=w281) -> ("States Out"=w280:string)  [unwired: 14 in]
      }
      frame "---------- Macro ----------" {
        # "Do not put any code in this frame.\n(It is a separator no-op. You can make a copy of this frame to create a new Macro frame)"
        n138 = call <vilib>:"Add State(s) to Queue__jki_lib_state_machine.vi"("State(s) in (\"\")"=w350) -> ("States Out"=w349:string)  [unwired: 14 in]
      }
      frame "Macro: Initialize" {
        w353 = FALSE  # debug mode
        w352 = "Data: Initialize\nInitialize Core Data\nUI: Initialize\nUI: Front Panel State >> Open\nUI: Front Panel State >> Open\nData: Initialize Top Level\nData: Initialize Lockin\nData: Reset >> True\nSweep: Initialize\nSweep: Simulate\nMacro: Exit"  # debug mode
        # "Initialization Macro\n(This is called once, when the VI starts)"
        n139 = Select(t=w352, s=w353, f="Data: Initialize\nInitialize Core Data\nUI: Initialize\nUI: Front Panel State >> Open\nData: Initialize Top Level\nData: Reset >> True\nMacro: Start Sweep\n") -> (s? t:f=w354:string)
        n140 = call <vilib>:"Add State(s) to Queue__jki_lib_state_machine.vi"("State(s) in Front (\"\")"=w354, "State(s) in (\"\")"=w358) -> ("States Out"=w357:string)  [unwired: 13 in]
      }
      frame "Macro: Start Sweep" {
        # "Do not put any code in this frame.\n(It is a separator no-op. You can make a copy of this frame to create a new Macro frame)"
        n141 = call <vilib>:"Add State(s) to Queue__jki_lib_state_machine.vi"("State(s) in Front (\"\")"="Sweep: Initialize\nAction: Move Delay Line >> Start\n//Action: Lockin >> Stop\nAction: Lockin Sampling\nSweep: Wait\nMeasure: Lockin >> Start\n//Action: Lockin >> Start\nMeasure: Delay Line\nAction: Move Delay Line >> End" ("State(s) in Front (\"\")"), "State(s) in (\"\")"=w363) -> ("States Out"=w362:string)  [unwired: 13 in]
      }
      frame "Macro: Sweeping" {
        # "Do not put any code in this frame.\n(It is a separator no-op. You can make a copy of this frame to create a new Macro frame)"
        n142 = call <vilib>:"Add State(s) to Queue__jki_lib_state_machine.vi"("State(s) in Front (\"\")"="Measure: Lockin\n//Measure: Temperature\nMeasure: Time\nMeasure: Delay Line\nUI: Update Graphs\nUI: Update Timer\nData: Reset >> False\nSweep: Check State\nData: Check Notifier" ("State(s) in Front (\"\")"), "State(s) in (\"\")"=w368) -> ("States Out"=w367:string)  [unwired: 13 in]
      }
      frame "Macro: Stop Sweep" {
        # "Do not put any code in this frame.\n(It is a separator no-op. You can make a copy of this frame to create a new Macro frame)"
        n143 = call <vilib>:"Add State(s) to Queue__jki_lib_state_machine.vi"("State(s) in Front (\"\")"="//Sweep: Stop\nUI: Update Graphs Final\nFile: Save\n//Action: Lockin >> Stop" ("State(s) in Front (\"\")"), "State(s) in (\"\")"=w373) -> ("States Out"=w372:string)  [unwired: 13 in]
      }
      frame "Macro: Exit" {
        # "Exit Macro\n(This is called once, when the VI exits)"
        n144 = Unbundle By Name(w380) -> ("Core.Close Panel on Exit?"=w379:bool)
        n145 = Select(t="UI: Front Panel State >> Close", s=w379, f="") -> (s? t:f=w376:string)
        n146 = call <vilib>:"Add State(s) to Queue__jki_lib_state_machine.vi"("State(s) in (\"\")"=w376, "State(s) at Back (\"\")"="Data: Cleanup\nExit") -> ("States Out"=w374:string)  [unwired: 13 in]
        n147 = call <vilib>:"Add State(s) to Queue__jki_lib_state_machine.vi"("State(s) in Front (\"\")"=w374, "State(s) in (\"\")"=w383) -> ("States Out"=w382:string)  [unwired: 13 in]
      }
      frame "---------- Sweep ----------" {
        # "Do not put any code in this frame.\n(It is a separator no-op. You can make a copy of this frame to create a new Macro frame)"
        n148 = call <vilib>:"Add State(s) to Queue__jki_lib_state_machine.vi"("State(s) in (\"\")"=w387) -> ("States Out"=w386:string)  [unwired: 14 in]
      }
      frame "Sweep: Initialize" {
        # "Do not put any code in this frame.\n(It is a separator no-op. You can make a copy of this frame to create a new Macro frame)"
        n149 = Unbundle By Name(w388) -> ("Instruments.Delay Line"=w398:refnum<class "Instrument.DelayLine.lvclass">)
        n150 = call-dynamic "Open.vi"("error in (no error)"=w397, "Instrument in"=w398) -> ("error out"=w393:errorcluster, "Instrument out"=w396:refnum<class "Instrument.DelayLine.lvclass">)  [unwired: 8 in]
        n151 = Subtract(x="Delay End (ps)", y="Delay Start (ps)") -> (x-y=w395:dbl)
        n152 = Absolute Value(x=w395) -> (abs(x)=w392:dbl)
        n153 = Divide(x=w392, y="Sweep Time (s)") -> (x/y=w394:dbl)
        n154 = Bundle By Name(cluster=w388, "Instruments.Delay Line"=w396, "Delay Range (ps)"=w392, "Delay Speed (ps/s)"=w394) -> (w399:T5)
        n155 = property on="Horizontal Progress Bar" class="Slide (strict)"("Scale.Maximum"="Delay End (ps)", "Scale.Minimum"="Delay Start (ps)") -> ()  [unwired: 2 in, 2 out]
        n156 = call <vilib>:"Add State(s) to Queue__jki_lib_state_machine.vi"("State(s) in (\"\")"=w401) -> ("States Out"=w400:string)  [unwired: 14 in]
      }
      frame "Sweep: Wait" {
        # "Do not put any code in this frame.\n(It is a separator no-op. You can make a copy of this frame to create a new Macro frame)"
        n157 = Multiply(x="Initial Wait (s)", y=u32 1000) -> (x*y=w403:u32)
        n158 = call <userlib>:"Wait (ms)__ogtk.vi"("error in (no error)"=w406, "milliseconds to wait"=w403) -> ("error out"=w405:errorcluster)  [unwired: 8 in, 1 out]
        n159 = call <vilib>:"Add State(s) to Queue__jki_lib_state_machine.vi"("State(s) in (\"\")"=w409) -> ("States Out"=w408:string)  [unwired: 14 in]
      }
      frame "Sweep: Stop" {
        # "#todo: is there a method to abort acquisition?"
        # "Do not put any code in this frame.\n(It is a separator no-op. You can make a copy of this frame to create a new Macro frame)"
        n160 = Unbundle By Name(w411) -> ()  [unwired: 1 out]
        n161 = call <vilib>:"Add State(s) to Queue__jki_lib_state_machine.vi"("State(s) in (\"\")"=w413) -> ("States Out"=w412:string)  [unwired: 14 in]
      }
      frame "Sweep: Check State" {
        # "Do not put any code in this frame.\n(It is a separator no-op. You can make a copy of this frame to create a new Macro frame)"
        n162 = Unbundle By Name(w419) -> ("delay line finish?"=w418:bool)
        n163 = Select(t="Macro: Sweeping\nMacro: Stop Sweep\nMacro: Exit" ("State(s) in Front (\"\")"), s=w418, f="") -> (s? t:f=w415:string)
        n164 = call <vilib>:"Add State(s) to Queue__jki_lib_state_machine.vi"("State(s) in Front (\"\")"=w415, "State(s) in (\"\")"=w421) -> ("States Out"=w420:string)  [unwired: 13 in]
      }
      frame "Sweep: Simulate" {
        # "Do not put any code in this frame.\n(It is a separator no-op. You can make a copy of this frame to create a new Macro frame)"
        n165 = Unbundle By Name(w423) -> ("Delay Speed (ps/s)"=w422:dbl)  [unwired: 1 out]
        n166 = while {
          tunnel: w422 -> [w436]
          i -> [w441]
          stop <- w439 stop-if-true
          n167 = Equal To 0?(x=w441) -> (x = 0?=w440:bool)
          n168 = local read "Delay Start (ps)"() -> (w438:dbl)
          n169 = call <userlib>:"MGI Milliseconds Since Last Reset.vi"("Reset (F)"=w440) -> ("ms"=w435:u32, "Error Out"=w429:errorcluster)  [unwired: 5 in]
          n170 = local read "Sweep Time (s)"() -> (w434:dbl)
          n171 = Divide(x=w435, y=1000.0) -> (x/y=w431:dbl)
          n172 = Multiply(x=w436, y=w431) -> (x*y=w432:dbl)
          n173 = call <userlib>:"MGI Milliseconds Since Last Call.vi"("Error In"=w429) -> ("ms"=w427:u32, "Error Out"=w428:errorcluster)  [unwired: 5 in]
          n174 = Add(x=w438, y=w432) -> (x+y=w437:dbl)
          n175 = local write "Elapsed Time (s)"(w431) -> ()
          n176 = Greater?(x=w431, y=w434) -> (0:w439:bool)
          n177 = local write "Refresh Time (ms)"(w427) -> ()
          n178 = call-poly <userlib>:"MGI Wait.vi"("ms"=u32 100, "Error In"=w428) -> ()  [unwired: 5 in, 1 out]
          n179 = local write "Horizontal Progress Bar"(w437) -> ()
          n180 = local write "Delay (ps)"(w437) -> ()
        }
        n181 = call <vilib>:"Add State(s) to Queue__jki_lib_state_machine.vi"("State(s) in (\"\")"=w426) -> ("States Out"=w425:string)  [unwired: 14 in]
      }
      frame "---------- Action ----------" {
        # "Do not put any code in this frame.\n(It is a separator no-op. You can make a copy of this frame to create a new Macro frame)"
        n182 = call <vilib>:"Add State(s) to Queue__jki_lib_state_machine.vi"("State(s) in (\"\")"=w445) -> ("States Out"=w444:string)  [unwired: 14 in]
      }
      frame "Action: Lockin" {
        # "Do not put any code in this frame.\n(It is a separator no-op. You can make a copy of this frame to create a new Macro frame)"
        n183 = Unbundle By Name(w448) -> ("Instruments.DAQ"=w451:refnum<class "Instrument.LockinAPI.lvclass">)
        n184 = case shown="\"Start\", Default" w452 {
          tunnel: w451 -> [w456 w461]
          tunnel: w450 -> [w458 w462]
          tunnel: [w457 w460] -> w449
          tunnel: [w455 w459] -> w447
          frame "Stop" {
            n185 = call-dynamic "waitStatusIdle.vi"("error in (no error)"=w458, "Instrument.LockinAPI in"=w456) -> ("error out"=w457:errorcluster, "Instrument.LockinAPI out"=w455:refnum<class "Instrument.LockinAPI.lvclass">)  [unwired: 8 in]
          }
          frame "Start", Default {
            n186 = call-dynamic "waitStatusSweepingStarted.vi"("error in (no error)"=w462, "Instrument.LockinAPI in"=w461) -> ("error out"=w460:errorcluster, "Instrument.LockinAPI out"=w459:refnum<class "Instrument.LockinAPI.lvclass">)  [unwired: 8 in]
          }
        }
        n187 = Bundle By Name(cluster=w448, "Instruments.DAQ"=w447) -> (w446:T5)
        n188 = call <vilib>:"Add State(s) to Queue__jki_lib_state_machine.vi"("State(s) in (\"\")"=w454) -> ("States Out"=w453:string)  [unwired: 14 in]
      }
      frame "Action: Lockin Sampling" {
        # "#todo: make sure Fs and N are in appropriate range"
        # "Do not put any code in this frame.\n(It is a separator no-op. You can make a copy of this frame to create a new Macro frame)"
        n189 = Unbundle By Name(w465) -> ("Instruments.DAQ"=w472:refnum<class "Instrument.LockinAPI.lvclass">)
        n190 = Multiply(x="Fs (S/s)", y="Lockin Refresh (s)") -> (x*y=w475:dbl)
        n191 = To Long Integer(number=w475) -> (32bit integer=w473:i32)
        n192 = call-dynamic "getSampling.vi"("error in (no error)"=w469, "Instrument.LockinAPI in"=w472) -> ("error out"=w468:errorcluster, "sampling"=w466:T8, "Instrument.LockinAPI out"=w471:refnum<class "Instrument.LockinAPI.lvclass">)  [unwired: 7 in]
        n193 = Bundle By Name(cluster=w466, "Fs"="Fs (S/s)", "#s"=w473) -> (w467:T8)
        n194 = Not Equal?(x=w466, y=w467) -> (x != y?=w470:bool)
        n195 = case shown="True" w470 {
          tunnel: w468 -> [w481 w486]
          tunnel: [w481 w485] -> w477
          tunnel: w471 -> [w480 w484]
          tunnel: w467 -> [_ w483]
          tunnel: [w480 w482] -> w463
          frame False {
          }
          frame True {
            n196 = call-dynamic "setSampling.vi"("error in (no error)"=w486, "sampling"=w483, "Instrument.LockinAPI in"=w484) -> ("error out"=w485:errorcluster, "Instrument.LockinAPI out"=w482:refnum<class "Instrument.LockinAPI.lvclass">)  [unwired: 7 in]
          }
        }
        n197 = Bundle By Name(cluster=w465, "Instruments.DAQ"=w463) -> (w464:T5)
        n198 = call <vilib>:"Add State(s) to Queue__jki_lib_state_machine.vi"("State(s) in (\"\")"=w479) -> ("States Out"=w478:string)  [unwired: 14 in]
      }
      frame "Action: Move Delay Line" {
        # "Do not put any code in this frame.\n(It is a separator no-op. You can make a copy of this frame to create a new Macro frame)"
        n199 = Unbundle By Name(w487) -> ("Instruments.Delay Line"=w496:refnum<class "Instrument.DelayLine.lvclass">, "Delay Speed (ps/s)"=w494:dbl)
        n200 = case shown="\"Start\", Default" w495 {
          tunnel: [w499 w502] -> w492
          tunnel: [1.0 ("Rate (ps/s)") w501] -> w493
          tunnel: w494 -> [_ w501]
          frame "Start", Default {
            n201 = local read "Delay Start (ps)"() -> (w499:dbl)
          }
          frame "End" {
            n202 = local read "Delay End (ps)"() -> (w502:dbl)
          }
        }
        n203 = call-dynamic "setDelay.vi"("error in (no error)"=w491, "Rate (ps/s)"=w493, "Delay (ps)"=w492, "Instrument.Delay in"=w496) -> ("error out"=w490:errorcluster, "Instrument.Delay out"=w489:refnum<class "Instrument.DelayLine.lvclass">)  [unwired: 6 in]
        n204 = Bundle By Name(cluster=w487, "Instruments.Delay Line"=w489) -> (w488:T5)
        n205 = call <vilib>:"Add State(s) to Queue__jki_lib_state_machine.vi"("State(s) in (\"\")"=w498) -> ("States Out"=w497:string)  [unwired: 14 in]
      }
      frame "Action: Close Delay Line" {
        # "Do not put any code in this frame.\n(It is a separator no-op. You can make a copy of this frame to create a new Macro frame)"
        n206 = Unbundle By Name(w505) -> ("Instruments.Delay Line"=w508:refnum<class "Instrument.DelayLine.lvclass">)
        n207 = call-dynamic "Close.vi"("error in (no error)"=w507, "Instrument in"=w508) -> ("error out"=w506:errorcluster, "Instrument out"=w504:refnum<class "Instrument.DelayLine.lvclass">)  [unwired: 8 in]
        n208 = Bundle By Name(cluster=w505, "Instruments.Delay Line"=w504) -> (w503:T5)
        n209 = call <vilib>:"Add State(s) to Queue__jki_lib_state_machine.vi"("State(s) in (\"\")"=w510) -> ("States Out"=w509:string)  [unwired: 14 in]
      }
      frame "---------- Measure ----------" {
        # "Template Separator\n(You can make a copy of, or modify, this frame)"
        n210 = call <vilib>:"Add State(s) to Queue__jki_lib_state_machine.vi"("State(s) in (\"\")"=w514) -> ("States Out"=w513:string)  [unwired: 14 in]
      }
      frame "Measure: Lockin" {
        # "Template Separator\n(You can make a copy of, or modify, this frame)"
        n211 = Unbundle By Name(w525) -> ("t0"=w519:timestamp, "AI Waveform (s)"=w523:waveform(dbl)[], "Instruments.DAQ"=w515:refnum<class "Instrument.LockinAPI.lvclass">)
        n212 = case shown="Default" w517 {
          tunnel: w523 -> [w532 w553]
          tunnel: [w532 w552] -> w522
          tunnel: [w534 w551] -> w521
          tunnel: w518 -> [w535 w550]
          tunnel: [w530 w546] -> w520
          tunnel: w515 -> [w536 w545]
          tunnel: w519 -> [_ w543]
          tunnel: [w528 w542] -> w516
          frame "Start" {
            n213 = for {
              N: 3 -> [_]
              tunnel: [w538] -> w529
              shift-right: [w539] -> w534
              shift-left: w535 -> [w540]
              shift-right: [w537] -> w528
              shift-left: w536 -> [w541]
              n214 = call-dynamic "waitNewWaveforms.vi"("error in (no error)"=w540, "Instrument.LockinAPI in"=w541) -> ("error out"=w539:errorcluster, "Newest AI Waveform"=w538:waveform(dbl)[], "Instrument.LockinAPI out"=w537:refnum<class "Instrument.LockinAPI.lvclass">)  [unwired: 7 in]
            }
            n215 = Index Array(array=w529) -> (element=w533:waveform(dbl))  [unwired: 1 in]
            n216 = Unbundle By Name(w533) -> ("t0"=w530:timestamp)
          }
          frame Default {
            n217 = call-dynamic "getAIwfm.vi"("error in (no error)"=w550, "Instrument.LockinAPI in"=w545) -> ("error out"=w549:errorcluster, "AI Waveform"=w544:waveform(dbl)[], "Instrument.LockinAPI out"=w542:refnum<class "Instrument.LockinAPI.lvclass">)  [unwired: 7 in]
            n218 = Index Array(array=w544) -> (element=w548:waveform(dbl))  [unwired: 1 in]
            n219 = Unbundle By Name(w548) -> ("t0"=w546:timestamp)
            n220 = Equal?(x=w546, y=w543) -> (x = y?=w547:bool)
            n221 = case shown="False" w547 {
              tunnel: w553 -> [w555 w572]
              tunnel: [w558 w572] -> w552
              tunnel: [w557 w573] -> w551
              tunnel: w549 -> [w556 w573]
              tunnel: w544 -> [w559 _]
              frame False {
                n222 = Array Size(array=w555) -> (size(s)=w554:i32)
                n223 = case shown="0" w554 {
                  tunnel: w559 -> [w561 w566]
                  tunnel: [w561 w565] -> w558
                  tunnel: [w560 w564] -> w557
                  tunnel: w556 -> [w560 w563]
                  tunnel: w555 -> [_ w562]
                  frame 0 {
                  }
                  frame Default {
                    n224 = for {
                      tunnel: w562 -> [w567] mode=indexing
                      tunnel: w566 -> [w571] mode=indexing
                      tunnel: [w570] -> w565 mode=indexing
                      tunnel: [w569] -> w564
                      tunnel: w563 -> [w568]
                      n225 = call-poly <vilib>:"Append Waveforms.vi"("error in (no error)"=w568, "waveform B"=w571, "waveform A"=w567) -> ("error out"=w569:errorcluster, "waveform out"=w570:waveform(dbl))  [unwired: 7 in]
                    }
                  }
                }
              }
              frame True {
              }
            }
          }
        }
        n226 = Bundle By Name(cluster=w525, "t0"=w520, "AI Waveform (s)"=w522, "Instruments.DAQ"=w516) -> (w524:T5)
        n227 = call <vilib>:"Add State(s) to Queue__jki_lib_state_machine.vi"("State(s) in (\"\")"=w527) -> ("States Out"=w526:string)  [unwired: 14 in]
      }
      frame "Measure: Temperature" {
        # "Your code here.\n(You can make a copy of, or modify, this frame)"
        n228 = Unbundle By Name(w582) -> ("C.E."=w577:refnum<class "Control Experiment.lvclass">, "Instruments.Temperature"=w584:refnum<class "Instrument.Cryostat.lvclass">)
        n229 = call-dynamic "getTemperature.vi"("error in (no error)"=w583, "Instrument.Cryostat in"=w584) -> ("error out"=w579:errorcluster, "Temperature (K)"=w578:dbl, "Instrument.Cryostat out"=w574:refnum<class "Instrument.Cryostat.lvclass">)  [unwired: 5 in, 2 out]
        "T (mK)" <- w578
        n230 = call "Append Dictionary Element.vi"("error in (no error)"=w579, "value"=w578, "key"="Temperature", "Control Experiment in"=w577) -> ("error out"=w576:errorcluster, "Control Experiment out"=w575:refnum<class "Control Experiment.lvclass">)  [unwired: 6 in]
        n231 = Bundle By Name(cluster=w582, "Instruments.Temperature"=w574, "Temperature"=w578, "C.E."=w575) -> (w581:T5)
        n232 = call <vilib>:"Add State(s) to Queue__jki_lib_state_machine.vi"("State(s) in (\"\")"=w586) -> ("States Out"=w585:string)  [unwired: 14 in]
      }
      frame "Measure: Time" {
        # "Your code here.\n(You can make a copy of, or modify, this frame)"
        n233 = Unbundle By Name(w605) -> ("reset"=w589:bool, "Elapsed Time"=w599:dbl[], "Absolute Time"=w593:dbl[], "C.E."=w603:refnum<class "Control Experiment.lvclass">)
        n234 = Get Date/Time In Seconds() -> (seconds since 1Jan1904=w595:timestamp)
        n235 = Select(t=2, s=w589, f=1) -> (s? t:f=w590:i32)
        n236 = for {
          N: w590 -> [_]
          tunnel: [w610] -> w597
          tunnel: w589 -> [w609]
          n237 = call <userlib>:"MGI Milliseconds Since Last Reset.vi"("Reset (F)"=w609) -> ("ms"=w610:u32)  [unwired: 5 in, 1 out]
        }
        n238 = To Double Precision Float(number=w595) -> (double precision float=w592:dbl)
        n239 = Divide(x=w597, y=u32 1000) -> (x/y=w596:dbl)
        n240 = call "Append Dictionary Element.vi"("error in (no error)"=w601, "value"=w592, "key"="Time", "Control Experiment in"=w603) -> ("error out"=w600:errorcluster, "Control Experiment out"=w604:refnum<class "Control Experiment.lvclass">)  [unwired: 6 in]
        n241 = Build Array (concatenate)(w593, w592) -> (w594:dbl[])
        n242 = Build Array (concatenate)(w599, w596) -> (w598:dbl[])
        n243 = Bundle By Name(cluster=w605, "Elapsed Time"=w598, "Absolute Time"=w594, "C.E."=w604) -> (w606:T5)
        n244 = call <vilib>:"Add State(s) to Queue__jki_lib_state_machine.vi"("State(s) in (\"\")"=w608) -> ("States Out"=w607:string)  [unwired: 14 in]
      }
      frame "Measure: Delay Line" {
        # "Template Separator\n(You can make a copy of, or modify, this frame)"
        n245 = Unbundle By Name(w624) -> ("Delay"=w618:dbl[], "C.E."=w619:refnum<class "Control Experiment.lvclass">, "Instruments.Delay Line"=w622:refnum<class "Instrument.DelayLine.lvclass">)
        n246 = call-dynamic "getDelay.vi"("error in (no error)"=w616, "Instrument.DelayLine in"=w622) -> ("error out"=w620:errorcluster, "delay (ps)"=w611:dbl, "Instrument.DelayLine out"=w612:refnum<class "Instrument.DelayLine.lvclass">, "Finished?"=w613:bool)  [unwired: 6 in]
        "Delay (ps)" <- w611
        "Horizontal Progress Bar" <- w611
        n247 = Build Array (concatenate)(w618, w611) -> (w617:dbl[])
        n248 = call "Append Dictionary Element.vi"("error in (no error)"=w620, "value"=w611, "key"="Delay", "Control Experiment in"=w619) -> ("error out"=w615:errorcluster, "Control Experiment out"=w621:refnum<class "Control Experiment.lvclass">)  [unwired: 6 in]
        n249 = Bundle By Name(cluster=w624, "Delay"=w617, "Instruments.Delay Line"=w612, "C.E."=w621, "delay line finish?"=w613) -> (w623:T5)
        n250 = call <vilib>:"Add State(s) to Queue__jki_lib_state_machine.vi"("State(s) in (\"\")"=w626) -> ("States Out"=w625:string)  [unwired: 14 in]
      }
      frame "---------- File ----------" {
        # "Template Separator\n(You can make a copy of, or modify, this frame)"
        n251 = call <vilib>:"Add State(s) to Queue__jki_lib_state_machine.vi"("State(s) in (\"\")"=w630) -> ("States Out"=w629:string)  [unwired: 14 in]
      }
      frame "File: Configure" {
        # "Template Separator\n(You can make a copy of, or modify, this frame)"
        n252 = call <vilib>:"Add State(s) to Queue__jki_lib_state_machine.vi"("State(s) in (\"\")"=w634) -> ("States Out"=w633:string)  [unwired: 14 in]
      }
      frame "File: Save" {
        # "Template Separator\n(You can make a copy of, or modify, this frame)"
        n253 = Unbundle By Name(w638) -> ("Execution:State"=w639:T6, "C.E."=w640:refnum<class "Control Experiment.lvclass">, "AI Waveform (ps)"=w641:waveform(dbl)[])
        n254 = for {
          tunnel: w640 -> [w684]
          tunnel: [w683] -> w646
          tunnel: [w682] -> w645
          tunnel: w643 -> [w667]
          tunnel: w641 -> [w662] mode=indexing
          tunnel: w643 -> [w656]
          tunnel: [w649] -> w642 mode=indexing
          i -> [w689]
          n255 = call-poly <vilib>:"Waveform to XY.vi"("error in (no error)"=w656, "Waveform in"=w662) -> ("error out"=w657:errorcluster, "XY-data out"=w660:cluster{"X-array":dbl[], "Y-array":dbl[]})  [unwired: 8 in]
          n256 = call-poly <vilib>:"FFT Power Spectrum and PSD.vi"("error in (no error)"=w656, "time signal"=w662) -> ("error out"=w651:errorcluster, "Power Spectrum / PSD"=w649:cluster{"f0":dbl, "df":dbl, "magnitude":dbl[]})  [unwired: 6 in, 2 out]
          n257 = Increment(x=w689) -> (x+1=w687:i32)
          n258 = call-poly <vilib>:"Get X and Y.vi"("error in (no error)"=w657, "XY-data"=w660) -> ("Y-array"=w658:dbl[], "X-array"=w659:dbl[])  [unwired: 6 in, 2 out]
          n259 = Format Into String(format string="Ch%d" ("wavenames"), w687) -> (resulting string=w668:string)  [unwired: 2 in, 1 out]
          n260 = Unbundle By Name(w649) -> ("f0"=w666:dbl, "df"=w665:dbl, "magnitude"=w664:dbl[])
          n261 = Concatenate Strings(w668, "_x" ("string")) -> (w676:string)
          n262 = call "Write Dictionary Element.vi"("error in (no error)"=w667, "value"=w659, "key"=w676, "Control Experiment in"=w684) -> ("error out"=w680:errorcluster, "Control Experiment out"=w681:refnum<class "Control Experiment.lvclass">)  [unwired: 6 in]
          n263 = To Time Stamp(1:w666) -> (0:w663:timestamp)
          n264 = Concatenate Strings(w668, "_y" ("string")) -> (w674:string)
          n265 = Bundle By Name("t0"=w663, "dt"=w665, "Y"=w664) -> (w650:waveform(dbl))  [unwired: 1 in]
          n266 = call "Write Dictionary Element.vi"("error in (no error)"=w680, "value"=w658, "key"=w674, "Control Experiment in"=w681) -> ("error out"=w661:errorcluster, "Control Experiment out"=w686:refnum<class "Control Experiment.lvclass">)  [unwired: 6 in]
          n267 = Concatenate Strings(w668, "_PS" ("string")) -> (w671:string)
          n268 = call-poly <vilib>:"Waveform to XY.vi"("error in (no error)"=w651, "Waveform in"=w650) -> ("error out"=w655:errorcluster, "XY-data out"=w654:cluster{"X-array":dbl[], "Y-array":dbl[]})  [unwired: 8 in]
          n269 = call-poly <vilib>:"Get X and Y.vi"("error in (no error)"=w655, "XY-data"=w654) -> ("Y-array"=w652:dbl[], "X-array"=w653:dbl[])  [unwired: 6 in, 2 out]
          n270 = Concatenate Strings(w671, "_x" ("string")) -> (w670:string)
          n271 = call "Write Dictionary Element.vi"("error in (no error)"=w661, "value"=w653, "key"=w670, "Control Experiment in"=w686) -> ("error out"=w678:errorcluster, "Control Experiment out"=w679:refnum<class "Control Experiment.lvclass">)  [unwired: 6 in]
          n272 = Concatenate Strings(w671, "_y" ("string")) -> (w669:string)
          n273 = call "Write Dictionary Element.vi"("error in (no error)"=w678, "value"=w652, "key"=w669, "Control Experiment in"=w679) -> ("error out"=w682:errorcluster, "Control Experiment out"=w683:refnum<class "Control Experiment.lvclass">)  [unwired: 6 in]
        }
        "Power Spectrum" <- w642
        n274 = call "Exec State to Append.vi"("Execution:State"=w639) -> ()  [unwired: 2 in, 1 out]
        n275 = call "Save Transport TDMS File.vi"("append?"=FALSE, "error in (no error)"=w645, "Control Experiment in"=w646) -> ("error out"=w644:errorcluster, "Control Experiment out"=w636:refnum<class "Control Experiment.lvclass">)  [unwired: 7 in]
        n276 = Bundle By Name(cluster=w638, "C.E."=w636) -> (w637:T5)
        n277 = call <vilib>:"Add State(s) to Queue__jki_lib_state_machine.vi"("State(s) in (\"\")"=w648) -> ("States Out"=w647:string)  [unwired: 14 in]
      }
      frame "File: JSON" {
        # "#todo: add save JSON stuff"
        # "Template Separator\n(You can make a copy of, or modify, this frame)"
        n278 = Unbundle By Name(w691) -> ()  [unwired: 1 out]
        n279 = call <vilib>:"Add State(s) to Queue__jki_lib_state_machine.vi"("State(s) in (\"\")"=w693) -> ("States Out"=w692:string)  [unwired: 14 in]
      }
    }
  }
  "error out" <- w3
  n280 = Unbundle By Name(w4) -> ("Transport"=→"Transport out":refnum<class "Transport.lvclass">)
